vi "rs232_build_visa_resource_name.vi"(7 "test mode":T1(ring), 9 "19052 COM settings":T2, 11 "19572 COM settings":T2) -> (1 "VISA Resource name 2":refnum<visa-resource-name>, 3 "VISA Resource name 1":refnum<visa-resource-name>)   [LabVIEW 2015]
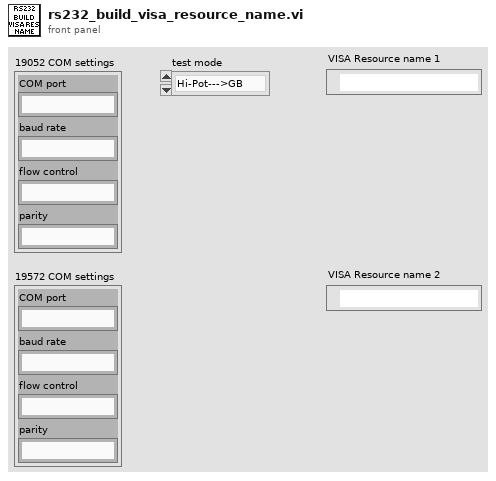
[diagram p1: front panel]
types:
  T1 = enum16{"Hi-Pot--->GB", "GB--->Hi-Pot", "Hi-Pot only", "GB only"}
  T2 = cluster{"COM port":string, "baud rate":string, "flow control":string, "parity":string}
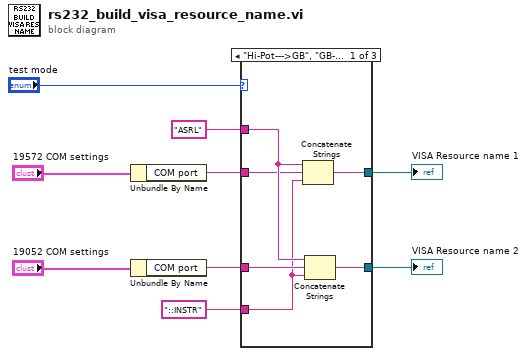
[diagram p0: block diagram]
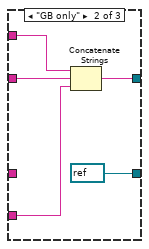
[diagram p2: hidden frame]
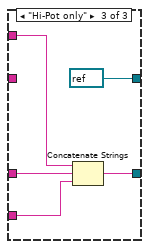
[diagram p3: hidden frame]
diagram:
  n1 = Unbundle By Name("19572 COM settings") -> ("COM port"=w6:string)
  n2 = Unbundle By Name("19052 COM settings") -> ("COM port"=w5:string)
  n3 = case shown="\"Hi-Pot--->GB\", \"GB--->Hi-Pot\"" "test mode" {
    tunnel: w6 -> [w10 w17 _]
    tunnel: w5 -> [w15 _ w25]
    tunnel: [w14 w20 refnum<visa-resource-name> refnum ("VISA res out 2")] -> w7
    tunnel: [w13 refnum<visa-resource-name> refnum ("VISA res out 2") w23] -> w4
    tunnel: "ASRL" -> [w12 w19 w22]
    tunnel: "::INSTR" -> [w11 w18 w21]
    frame "Hi-Pot--->GB", "GB--->Hi-Pot" {
      n4 = Concatenate Strings(w12, w10, w11) -> (w14:string)
      n5 = Concatenate Strings(w12, w15, w11) -> (w13:string)
    }
    frame "GB only" {
      n6 = Concatenate Strings(w19, w17, w18) -> (w20:string)
    }
    frame "Hi-Pot only" {
      n7 = Concatenate Strings(w22, w25, w21) -> (w23:string)
    }
  }
  "VISA Resource name 2" <- w4
  "VISA Resource name 1" <- w7
